vi "Initialize.vi"(6 "Default return":variant, 7 "reader buffer size":i32=4096, 8 "error in (no error)":errorcluster, 10 "writer url":string, 11 "reader name":string) -> (0 "error out":errorcluster, 3 "NetworkStreamWriter out":refnum<class "NetworkStreamReader.lvclass">)   [LabVIEW 2013, in "NetworkStreamReader.lvclass"]
doc: "Instantiates an instance of the NetworkStreamReader class. A NetworkStreamReader Object is a wrapper around the LabVIEW Network Stream Reader. The wrapper provides a reconnectable connection and separates reads from the Object from network communication. As with network streams, the writer url on the reader or the reader url on the writer must be given in order to establish the connection. The Object will read data from the network stream at a fixed rate in the background. This allows an application to read data from the Object in time-critical loops, as network communication occurs in a separate loop in the background.\n\n<b>It is critical that all initialized NetworkStreamReader Objects are closed with the Close method.</b> This method signals the background process to stop. If the Close method is not called, the background process will continue to run on the host computer. For this reason, <b>do not abort an application which uses NetworkStreamReader Objects.</b>\n\nNote that <b>the NetworkStreamReader Object is implemented to work by-reference</b>, meaning that copies of an initialized NetworkStreamReader Object will write to the same network stream internally.\n\nJared Kirschner, 2012."
uses:
  NetworkStreamReader.lvclass
  ReaderParameters.ctl
  Shared/TimeStampedMessage.ctl
  Shared/TimeStampedMessageQueue.ctl
  NetworkStreamReader.lvclass/NetworkStreamReader.ctl
  ReaderDaemon.vi
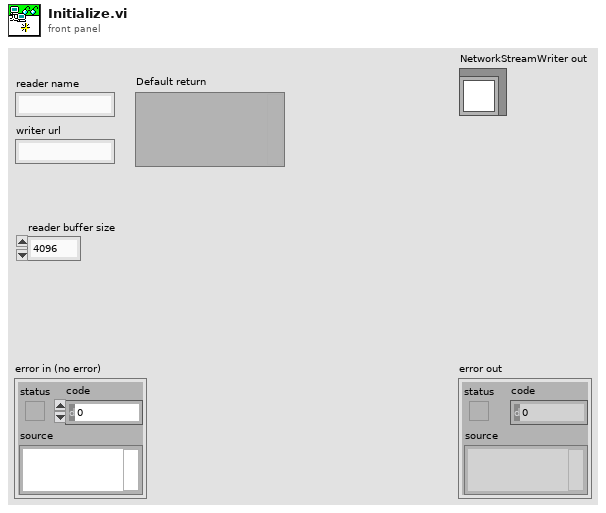
[diagram p1: front panel]
types:
  T1 = typedef "TimeStampedMessageQueue.ctl" = refnum<queue>
  T2 = typedef "TimeStampedMessage.ctl" = cluster{"Data":variant, "Time Stamp":timestamp}
  T3 = typedef "NetworkStreamReader.lvclass/ReaderParameters.ctl" = cluster{"reader name":string, "writer url":string, "reader buffer size":i32}
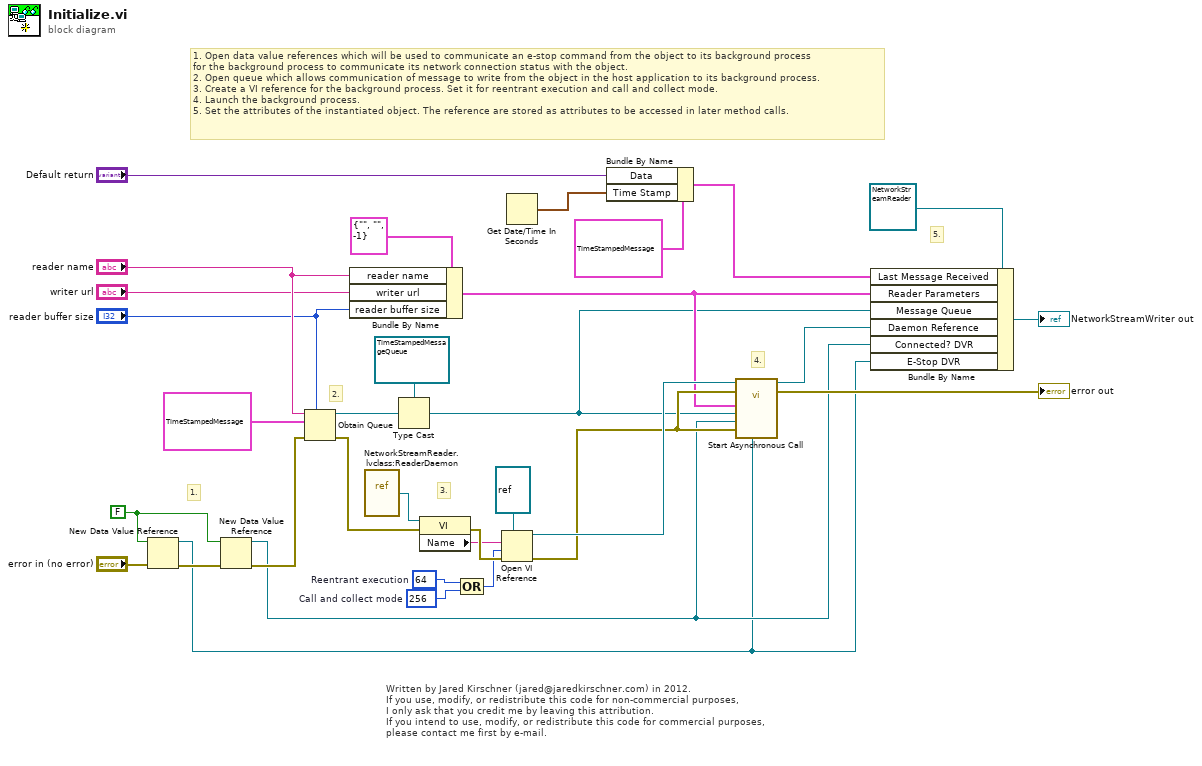
[diagram p0: block diagram]
diagram:
  w17 = FALSE
  w25 = 64  # Reentrant execution
  w26 = 256  # Call and collect mode
  # "5."
  # "4."
  # "3."
  # "2."
  # "1."
  # "1. Open data value references which will be used to communicate an e-stop command from the object to its background process\nfor the background process to communicate its network connection status with the object.\n2. Open queue which allows communication of message to write from the object in the host application to its background process.\n3. Create a VI reference for the background process. Set it for reentrant execution and call and collect mode.\n4. Launch the background process.\n5. Set the attributes of the instantiated object. The reference are stored as attributes to be accessed in later method calls."
  # "Written by Jared Kirschner (jared@jaredkirschner.com) in 2012.\nIf you use, modify, or redistribute this code for non-commercial purposes,\nI only ask that you credit me by leaving this attribution.\nIf you intend to use, modify, or redistribute this code for commercial purposes,\nplease contact me first by e-mail."
  n1 = New Data Value Reference(data value=w17, error in="error in (no error)") -> (data value reference=w8:refnum<data-value>, error out=w15:errorcluster)
  n2 = New Data Value Reference(data value=w17, error in=w15) -> (data value reference=w9:refnum<data-value>, error out=w14:errorcluster)
  n3 = Obtain Queue(max queue size (-1, unlimited)="reader buffer size", name (unnamed)="reader name", element data type=T2 {"Data"=variant, "Time Stamp"=timestamp(0 s since 1904-01-01)}, error in (no error)=w14) -> (queue out=w23:refnum<queue>, error out=w13:errorcluster)  [unwired: 1 in, 1 out]
  n4 = Bundle By Name(cluster=T3 {"reader name"="", "writer url"="", "reader buffer size"=-1} ("Reader Parameters"), "reader name"="reader name", "writer url"="writer url", "reader buffer size"="reader buffer size") -> (w6:T3)
  n5 = vi-ref "NetworkStreamReader.lvclass:ReaderDaemon.vi"() -> (w28:refnum<vi>)
  n6 = Type Cast(type=T1 refnum ("Variant Queue"), x=w23) -> (*(type *) &x=w2:T1)
  n7 = property class="VI"(reference=w28, error in=w13) -> (error out=w31:errorcluster, "Name"=w29:string)  [unwired: 1 out]
  n8 = Compound Arithmetic op=OR(w25, w26) -> (w24:i32)
  n9 = Open VI Reference(type specifier VI Refnum (for type only)=refnum<vi> refnum, vi path=w29, options=w24, error in (no error)=w31) -> (vi reference=w27:refnum<vi>, error out=w12:errorcluster)  [unwired: 2 in]
  n10 = Get Date/Time In Seconds() -> (seconds since 1Jan1904=w5:timestamp)
  n11 = Bundle By Name(cluster=T2 {"Data"=variant, "Time Stamp"=timestamp(0 s since 1904-01-01)} ("element data type"), "Data"="Default return", "Time Stamp"=w5) -> (w3:T2)
  n12 = call-by-ref "Start Asynchronous Call"(reference=w27, error in=w12, "E-Stop DVR"=w8, 8:"error in (no error)"=w12, "Connected? DVR"=w9, "Variant Queue"=w2, "Reader Parameters"=w6) -> (reference out=w10:refnum<vi>, error out=→"error out":errorcluster)  [unwired: 6 in, 1 out]
  n13 = Bundle By Name(cluster=refnum<class "NetworkStreamReader.lvclass"> refnum ("NetworkStreamWriter out"), "Last Message Received"=w3, "Reader Parameters"=w6, "Message Queue"=w2, "Daemon Reference"=w10, "Connected? DVR"=w9, "E-Stop DVR"=w8) -> (→"NetworkStreamWriter out":refnum<class "NetworkStreamReader.lvclass">)
